vi "(Delta)^2_RH_v2 - Copy.vi"() -> ()   [LabVIEW 2019]
uses:
  <vilib>/Analysis/baseanly.llb/Mean (DBL).vi
  Components/DeltaRamp_globals.vi
  Components/B_Globals.vi
  Components/Global 2.vi
  <vilib>/Analysis/NI_AALBase.lvlib
panel:
  out "Arm 2":bool
  out "Arm 1":bool
  in  "Graphing":string(combo)
  in  "I_2":dbl
  out "T 3":cluster{"X":dbl[], "Y":dbl[]}[](graph)=[{"X"=[1.6944000000000004, 1.6942999999999993, 1.6944, 1.6942999999999993, 1.6942000000000002, 1.6943, 1.6941999999999995, 1.6943, 1.6942000000000002, 1.6943, 1.6944, 1.6942000000000006, 1.6942999999999993, 1.6944, 1.6942999999999988, 1.6942000000000002, 1.6942999999999993, 1.6942000000000002, 1.6940999999999997, 1.6942000000000002, 1.6944000000000008, 1.6945, 1.6944000000000008, 1.6942999999999993, 1.6944000000000008, 1.6942999999999988, 1.6944000000000004, 1.694299999999999, 1.6945, 1.6945999999999999, 1.6945, 1.6944000000000012, 1.694299999999999, 1.6944, 1.6945, 1.6944000000000008, 1.6945000000000006, 1.6946000000000003, 1.6944999999999995, 1.6945999999999999, 1.6944000000000004, 1.6945, 1.6945999999999999, 1.6945, 1.6944, 1.6945000000000017, 1.6946000000000003, 1.6947000000000005, 1.6948000000000003, 1.6949000000000003, 1.6948000000000003, 1.6947000000000008, 1.6946000000000008, 1.6947000000000005, 1.6948000000000005, 1.6947000000000003, 1.6946, 1.6947000000000008, 1.6945999999999999, 1.6947000000000005, 1.6946000000000006, 1.6947000000000008, 1.6948000000000003, 1.6946999999999992, 1.6948000000000003, 1.6947000000000005, 1.6948000000000005, 1.6949000000000003, 1.6948000000000005, 1.694899999999999, 1.6951, 1.695, 1.6949000000000003, 1.6948000000000003, 1.694899999999999, 1.695, 1.6948999999999992, 1.6948000000000003, 1.6947000000000008, 1.6949000000000003, 1.695, 1.6949000000000003, 1.695, 1.6949000000000003, 1.6948000000000003, 1.6949000000000003, 1.6948000000000003, 1.6949000000000003, 1.695, 1.6951, 1.6952, 1.6951, 1.6952, 1.6951, 1.695, 1.6948000000000003, 1.6949000000000003, 1.695], "Y"=[nan, nan, nan, nan, nan, nan, nan, nan, nan, nan, nan, nan, nan, nan, nan, nan, nan, nan, nan, nan, nan, nan, nan, nan, nan, nan, nan, nan, nan, nan, nan, nan, nan, nan, nan, nan, nan, nan, nan, nan, nan, nan, nan, nan, nan, nan, nan, nan, nan, nan, nan, nan, nan, nan, nan, nan, nan, nan, nan, nan, nan, nan, nan, nan, nan, nan, nan, nan, nan, nan, nan, nan, nan, nan, nan, nan, nan, nan, nan, nan, nan, nan, nan, nan, nan, nan, nan, nan, nan, nan, nan, nan, nan, nan, nan, nan, nan, nan]}, {"X"=[1.6944000000000004, 1.6942999999999993, 1.6944, 1.6942999999999993, 1.6942000000000002, 1.6943, 1.6941999999999995, 1.6943, 1.6942000000000002, 1.6943, 1.6944, 1.6942000000000006, 1.6942999999999993, 1.6944, 1.6942999999999988, 1.6942000000000002, 1.6942999999999993, 1.6942000000000002, 1.6940999999999997, 1.6942000000000002, 1.6944000000000008, 1.6945, 1.6944000000000008, 1.6942999999999993, 1.6944000000000008, 1.6942999999999988, 1.6944000000000004, 1.694299999999999, 1.6945, 1.6945999999999999, 1.6945, 1.6944000000000012, 1.694299999999999, 1.6944, 1.6945, 1.6944000000000008, 1.6945000000000006, 1.6946000000000003, 1.6944999999999995, 1.6945999999999999, 1.6944000000000004, 1.6945, 1.6945999999999999, 1.6945, 1.6944, 1.6945000000000017, 1.6946000000000003, 1.6947000000000005, 1.6948000000000003, 1.6949000000000003, 1.6948000000000003, 1.6947000000000008, 1.6946000000000008, 1.6947000000000005, 1.6948000000000005, 1.6947000000000003, 1.6946, 1.6947000000000008, 1.6945999999999999, 1.6947000000000005, 1.6946000000000006, 1.6947000000000008, 1.6948000000000003, 1.6946999999999992, 1.6948000000000003, 1.6947000000000005, 1.6948000000000005, 1.6949000000000003, 1.6948000000000005, 1.694899999999999, 1.6951, 1.695, 1.6949000000000003, 1.6948000000000003, 1.694899999999999, 1.695, 1.6948999999999992, 1.6948000000000003, 1.6947000000000008, 1.6949000000000003, 1.695, 1.6949000000000003, 1.695, 1.6949000000000003, 1.6948000000000003, 1.6949000000000003, 1.6948000000000003, 1.6949000000000003, 1.695, 1.6951, 1.6952, 1.6951, 1.6952, 1.6951, 1.695, 1.6948000000000003, 1.6949000000000003, 1.695], "Y"=[19.228962826666663, 19.229748019999995, 19.227549399999997, 19.232509233333335, 19.230370125, 19.231082114285716, 19.231533643749998, 19.2332894875, 19.234548728000004, 19.23138665, 19.23452267142857, 19.233269309999994, 19.2297025, 19.228221342857143, 19.230086174193545, 19.2305463125, 19.22998058125, 19.234866695833333, 19.232316606250002, 19.2317453, 19.234343370833333, 19.232386587500002, 19.231900426086955, 19.23144366666667, 19.23149760833333, 19.229992476666673, 19.230156412500005, 19.23336701304348, 19.2296826625, 19.232198475, 19.2310109125, 19.231653921794866, 19.228340475000003, 19.2295796875, 19.229462228571432, 19.2302099, 19.22956034666667, 19.233207449999995, 19.23203613684211, 19.232299549999997, 19.2309091125, 19.229504266666666, 19.230617525, 19.230744125, 19.231113187500004, 19.22967935322581, 19.230101100000002, 19.230308512500002, 19.228578285714285, 19.233646177777775, 19.231167942857144, 19.23003209333333, 19.23084153157895, 19.22980882222222, 19.23070347608696, 19.227994165217392, 19.230754216666664, 19.229694923529415, 19.23029495, 19.229152924999998, 19.231262049999998, 19.23127544, 19.231315600000002, 19.230833448717952, 19.229475299999997, 19.23220135, 19.229062404918036, 19.230352887500004, 19.23155630625, 19.23113153225807, 19.234514033333337, 19.23535129285714, 19.23361205, 19.232085249999997, 19.232065674999998, 19.230572292857143, 19.230861596666667, 19.2296080625, 19.231095506666673, 19.230930925, 19.230720785714286, 19.230639773333333, 19.231475349999997, 19.23118514, 19.2300918125, 19.232860700000003, 19.2284774875, 19.2328781875, 19.2326205, 19.230885100000002, 19.231523024999998, 19.229335787500002, 19.231723528571425, 19.231652535294117, 19.2325406, 19.22911017142857, 19.23088324375, 19.231545675]}] caption="XY Graph"
  out "T 2":cluster{"X":dbl[], "Y":dbl[]}[](graph)=[{"X"=[1.6944000000000004, 1.6942999999999993, 1.6944, 1.6942999999999993, 1.6942000000000002, 1.6943, 1.6941999999999995, 1.6943, 1.6942000000000002, 1.6943, 1.6944, 1.6942000000000006, 1.6942999999999993, 1.6944, 1.6942999999999988, 1.6942000000000002, 1.6942999999999993, 1.6942000000000002, 1.6940999999999997, 1.6942000000000002, 1.6944000000000008, 1.6945, 1.6944000000000008, 1.6942999999999993, 1.6944000000000008, 1.6942999999999988, 1.6944000000000004, 1.694299999999999, 1.6945, 1.6945999999999999, 1.6945, 1.6944000000000012, 1.694299999999999, 1.6944, 1.6945, 1.6944000000000008, 1.6945000000000006, 1.6946000000000003, 1.6944999999999995, 1.6945999999999999, 1.6944000000000004, 1.6945, 1.6945999999999999, 1.6945, 1.6944, 1.6945000000000017, 1.6946000000000003, 1.6947000000000005, 1.6948000000000003, 1.6949000000000003, 1.6948000000000003, 1.6947000000000008, 1.6946000000000008, 1.6947000000000005, 1.6948000000000005, 1.6947000000000003, 1.6946, 1.6947000000000008, 1.6945999999999999, 1.6947000000000005, 1.6946000000000006, 1.6947000000000008, 1.6948000000000003, 1.6946999999999992, 1.6948000000000003, 1.6947000000000005, 1.6948000000000005, 1.6949000000000003, 1.6948000000000005, 1.694899999999999, 1.6951, 1.695, 1.6949000000000003, 1.6948000000000003, 1.694899999999999, 1.695, 1.6948999999999992, 1.6948000000000003, 1.6947000000000008, 1.6949000000000003, 1.695, 1.6949000000000003, 1.695, 1.6949000000000003, 1.6948000000000003, 1.6949000000000003, 1.6948000000000003, 1.6949000000000003, 1.695, 1.6951, 1.6952, 1.6951, 1.6952, 1.6951, 1.695, 1.6948000000000003, 1.6949000000000003, 1.695], "Y"=[nan, nan, nan, nan, nan, nan, nan, nan, nan, nan, nan, nan, nan, nan, nan, nan, nan, nan, nan, nan, nan, nan, nan, nan, nan, nan, nan, nan, nan, nan, nan, nan, nan, nan, nan, nan, nan, nan, nan, nan, nan, nan, nan, nan, nan, nan, nan, nan, nan, nan, nan, nan, nan, nan, nan, nan, nan, nan, nan, nan, nan, nan, nan, nan, nan, nan, nan, nan, nan, nan, nan, nan, nan, nan, nan, nan, nan, nan, nan, nan, nan, nan, nan, nan, nan, nan, nan, nan, nan, nan, nan, nan, nan, nan, nan, nan, nan, nan]}, {"X"=[1.6944000000000004, 1.6942999999999993, 1.6944, 1.6942999999999993, 1.6942000000000002, 1.6943, 1.6941999999999995, 1.6943, 1.6942000000000002, 1.6943, 1.6944, 1.6942000000000006, 1.6942999999999993, 1.6944, 1.6942999999999988, 1.6942000000000002, 1.6942999999999993, 1.6942000000000002, 1.6940999999999997, 1.6942000000000002, 1.6944000000000008, 1.6945, 1.6944000000000008, 1.6942999999999993, 1.6944000000000008, 1.6942999999999988, 1.6944000000000004, 1.694299999999999, 1.6945, 1.6945999999999999, 1.6945, 1.6944000000000012, 1.694299999999999, 1.6944, 1.6945, 1.6944000000000008, 1.6945000000000006, 1.6946000000000003, 1.6944999999999995, 1.6945999999999999, 1.6944000000000004, 1.6945, 1.6945999999999999, 1.6945, 1.6944, 1.6945000000000017, 1.6946000000000003, 1.6947000000000005, 1.6948000000000003, 1.6949000000000003, 1.6948000000000003, 1.6947000000000008, 1.6946000000000008, 1.6947000000000005, 1.6948000000000005, 1.6947000000000003, 1.6946, 1.6947000000000008, 1.6945999999999999, 1.6947000000000005, 1.6946000000000006, 1.6947000000000008, 1.6948000000000003, 1.6946999999999992, 1.6948000000000003, 1.6947000000000005, 1.6948000000000005, 1.6949000000000003, 1.6948000000000005, 1.694899999999999, 1.6951, 1.695, 1.6949000000000003, 1.6948000000000003, 1.694899999999999, 1.695, 1.6948999999999992, 1.6948000000000003, 1.6947000000000008, 1.6949000000000003, 1.695, 1.6949000000000003, 1.695, 1.6949000000000003, 1.6948000000000003, 1.6949000000000003, 1.6948000000000003, 1.6949000000000003, 1.695, 1.6951, 1.6952, 1.6951, 1.6952, 1.6951, 1.695, 1.6948000000000003, 1.6949000000000003, 1.695], "Y"=[19.228962826666663, 19.229748019999995, 19.227549399999997, 19.232509233333335, 19.230370125, 19.231082114285716, 19.231533643749998, 19.2332894875, 19.234548728000004, 19.23138665, 19.23452267142857, 19.233269309999994, 19.2297025, 19.228221342857143, 19.230086174193545, 19.2305463125, 19.22998058125, 19.234866695833333, 19.232316606250002, 19.2317453, 19.234343370833333, 19.232386587500002, 19.231900426086955, 19.23144366666667, 19.23149760833333, 19.229992476666673, 19.230156412500005, 19.23336701304348, 19.2296826625, 19.232198475, 19.2310109125, 19.231653921794866, 19.228340475000003, 19.2295796875, 19.229462228571432, 19.2302099, 19.22956034666667, 19.233207449999995, 19.23203613684211, 19.232299549999997, 19.2309091125, 19.229504266666666, 19.230617525, 19.230744125, 19.231113187500004, 19.22967935322581, 19.230101100000002, 19.230308512500002, 19.228578285714285, 19.233646177777775, 19.231167942857144, 19.23003209333333, 19.23084153157895, 19.22980882222222, 19.23070347608696, 19.227994165217392, 19.230754216666664, 19.229694923529415, 19.23029495, 19.229152924999998, 19.231262049999998, 19.23127544, 19.231315600000002, 19.230833448717952, 19.229475299999997, 19.23220135, 19.229062404918036, 19.230352887500004, 19.23155630625, 19.23113153225807, 19.234514033333337, 19.23535129285714, 19.23361205, 19.232085249999997, 19.232065674999998, 19.230572292857143, 19.230861596666667, 19.2296080625, 19.231095506666673, 19.230930925, 19.230720785714286, 19.230639773333333, 19.231475349999997, 19.23118514, 19.2300918125, 19.232860700000003, 19.2284774875, 19.2328781875, 19.2326205, 19.230885100000002, 19.231523024999998, 19.229335787500002, 19.231723528571425, 19.231652535294117, 19.2325406, 19.22911017142857, 19.23088324375, 19.231545675]}] caption="XY Graph"
  in  "Clear Paths":bool
  out "Remote Inherit Path":path=path "C:/User Data/hlb54/210307/RH_T=35p00K.txt"
  out "Remote Directory":path=path "C:/User Data/hlb54/210307"
  out "Last Saved":path=path "C:/User Data/gy251/20210308 Nb2p5-EuS30-Nb3_C/Rxx_9-10-11-12/RT_10uA_1.txt"
  out "Remote_Save_String [This is the important one!]":string="RH_T=35p00K.txt"
  in  "L1 ID":string="56A"
  in  "D1 ID":string="GY1C"
  out "R2":dbl=19.2284241
  in  "D2_use":bool=TRUE
  in  "D1_use":bool
  in  "D2":refnum<visa-resource-name>="GPIB1::22::INSTR" caption="Back"
  in  "Front":refnum<visa-resource-name>="GPIB1::20::INSTR"
  out "B_set [T]":dbl=3.0
  in  "Reading Delay [ms]":i32=20 min=5
  in  "RW Delay":i32=5
  out "Exec Time [ms]":u32=39
  in  "B/T":bool=TRUE
  in  "Smart Avs":bool=TRUE
  in  "Points":dbl=1.0
  out "PpP":dbl=8.0
  in  "Combo Box":string(combo)="Temp"
  in  "Save":bool
  in  "Abort":bool
  out "B [T]":dbl=2.98877
  in  "Arm":bool
  in  "Measure":bool
  in  "I_1":dbl=5e-05
  out "T":cluster{"X":dbl[], "Y":dbl[]}[](graph)=[{"X"=[1.6944000000000004, 1.6942999999999993, 1.6944, 1.6942999999999993, 1.6942000000000002, 1.6943, 1.6941999999999995, 1.6943, 1.6942000000000002, 1.6943, 1.6944, 1.6942000000000006, 1.6942999999999993, 1.6944, 1.6942999999999988, 1.6942000000000002, 1.6942999999999993, 1.6942000000000002, 1.6940999999999997, 1.6942000000000002, 1.6944000000000008, 1.6945, 1.6944000000000008, 1.6942999999999993, 1.6944000000000008, 1.6942999999999988, 1.6944000000000004, 1.694299999999999, 1.6945, 1.6945999999999999, 1.6945, 1.6944000000000012, 1.694299999999999, 1.6944, 1.6945, 1.6944000000000008, 1.6945000000000006, 1.6946000000000003, 1.6944999999999995, 1.6945999999999999, 1.6944000000000004, 1.6945, 1.6945999999999999, 1.6945, 1.6944, 1.6945000000000017, 1.6946000000000003, 1.6947000000000005, 1.6948000000000003, 1.6949000000000003, 1.6948000000000003, 1.6947000000000008, 1.6946000000000008, 1.6947000000000005, 1.6948000000000005, 1.6947000000000003, 1.6946, 1.6947000000000008, 1.6945999999999999, 1.6947000000000005, 1.6946000000000006, 1.6947000000000008, 1.6948000000000003, 1.6946999999999992, 1.6948000000000003, 1.6947000000000005, 1.6948000000000005, 1.6949000000000003, 1.6948000000000005, 1.694899999999999, 1.6951, 1.695, 1.6949000000000003, 1.6948000000000003, 1.694899999999999, 1.695, 1.6948999999999992, 1.6948000000000003, 1.6947000000000008, 1.6949000000000003, 1.695, 1.6949000000000003, 1.695, 1.6949000000000003, 1.6948000000000003, 1.6949000000000003, 1.6948000000000003, 1.6949000000000003, 1.695, 1.6951, 1.6952, 1.6951, 1.6952, 1.6951, 1.695, 1.6948000000000003, 1.6949000000000003, 1.695], "Y"=[nan, nan, nan, nan, nan, nan, nan, nan, nan, nan, nan, nan, nan, nan, nan, nan, nan, nan, nan, nan, nan, nan, nan, nan, nan, nan, nan, nan, nan, nan, nan, nan, nan, nan, nan, nan, nan, nan, nan, nan, nan, nan, nan, nan, nan, nan, nan, nan, nan, nan, nan, nan, nan, nan, nan, nan, nan, nan, nan, nan, nan, nan, nan, nan, nan, nan, nan, nan, nan, nan, nan, nan, nan, nan, nan, nan, nan, nan, nan, nan, nan, nan, nan, nan, nan, nan, nan, nan, nan, nan, nan, nan, nan, nan, nan, nan, nan, nan]}, {"X"=[1.6944000000000004, 1.6942999999999993, 1.6944, 1.6942999999999993, 1.6942000000000002, 1.6943, 1.6941999999999995, 1.6943, 1.6942000000000002, 1.6943, 1.6944, 1.6942000000000006, 1.6942999999999993, 1.6944, 1.6942999999999988, 1.6942000000000002, 1.6942999999999993, 1.6942000000000002, 1.6940999999999997, 1.6942000000000002, 1.6944000000000008, 1.6945, 1.6944000000000008, 1.6942999999999993, 1.6944000000000008, 1.6942999999999988, 1.6944000000000004, 1.694299999999999, 1.6945, 1.6945999999999999, 1.6945, 1.6944000000000012, 1.694299999999999, 1.6944, 1.6945, 1.6944000000000008, 1.6945000000000006, 1.6946000000000003, 1.6944999999999995, 1.6945999999999999, 1.6944000000000004, 1.6945, 1.6945999999999999, 1.6945, 1.6944, 1.6945000000000017, 1.6946000000000003, 1.6947000000000005, 1.6948000000000003, 1.6949000000000003, 1.6948000000000003, 1.6947000000000008, 1.6946000000000008, 1.6947000000000005, 1.6948000000000005, 1.6947000000000003, 1.6946, 1.6947000000000008, 1.6945999999999999, 1.6947000000000005, 1.6946000000000006, 1.6947000000000008, 1.6948000000000003, 1.6946999999999992, 1.6948000000000003, 1.6947000000000005, 1.6948000000000005, 1.6949000000000003, 1.6948000000000005, 1.694899999999999, 1.6951, 1.695, 1.6949000000000003, 1.6948000000000003, 1.694899999999999, 1.695, 1.6948999999999992, 1.6948000000000003, 1.6947000000000008, 1.6949000000000003, 1.695, 1.6949000000000003, 1.695, 1.6949000000000003, 1.6948000000000003, 1.6949000000000003, 1.6948000000000003, 1.6949000000000003, 1.695, 1.6951, 1.6952, 1.6951, 1.6952, 1.6951, 1.695, 1.6948000000000003, 1.6949000000000003, 1.695], "Y"=[19.228962826666663, 19.229748019999995, 19.227549399999997, 19.232509233333335, 19.230370125, 19.231082114285716, 19.231533643749998, 19.2332894875, 19.234548728000004, 19.23138665, 19.23452267142857, 19.233269309999994, 19.2297025, 19.228221342857143, 19.230086174193545, 19.2305463125, 19.22998058125, 19.234866695833333, 19.232316606250002, 19.2317453, 19.234343370833333, 19.232386587500002, 19.231900426086955, 19.23144366666667, 19.23149760833333, 19.229992476666673, 19.230156412500005, 19.23336701304348, 19.2296826625, 19.232198475, 19.2310109125, 19.231653921794866, 19.228340475000003, 19.2295796875, 19.229462228571432, 19.2302099, 19.22956034666667, 19.233207449999995, 19.23203613684211, 19.232299549999997, 19.2309091125, 19.229504266666666, 19.230617525, 19.230744125, 19.231113187500004, 19.22967935322581, 19.230101100000002, 19.230308512500002, 19.228578285714285, 19.233646177777775, 19.231167942857144, 19.23003209333333, 19.23084153157895, 19.22980882222222, 19.23070347608696, 19.227994165217392, 19.230754216666664, 19.229694923529415, 19.23029495, 19.229152924999998, 19.231262049999998, 19.23127544, 19.231315600000002, 19.230833448717952, 19.229475299999997, 19.23220135, 19.229062404918036, 19.230352887500004, 19.23155630625, 19.23113153225807, 19.234514033333337, 19.23535129285714, 19.23361205, 19.232085249999997, 19.232065674999998, 19.230572292857143, 19.230861596666667, 19.2296080625, 19.231095506666673, 19.230930925, 19.230720785714286, 19.230639773333333, 19.231475349999997, 19.23118514, 19.2300918125, 19.232860700000003, 19.2284774875, 19.2328781875, 19.2326205, 19.230885100000002, 19.231523024999998, 19.229335787500002, 19.231723528571425, 19.231652535294117, 19.2325406, 19.22911017142857, 19.23088324375, 19.231545675]}] caption="XY Graph"
  in  "Reset":bool
  out "Spl T [K]":dbl=1.6949
  out "R1 [Ohm]":dbl=nan
  # "Use?"
  # "Armed?"
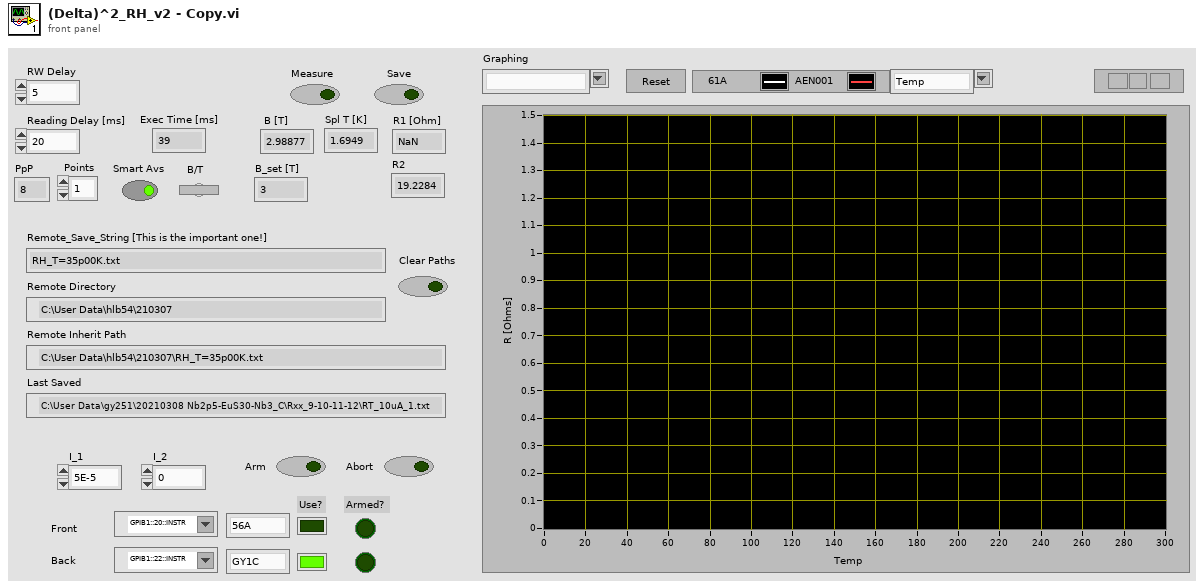
[diagram p1: front panel]
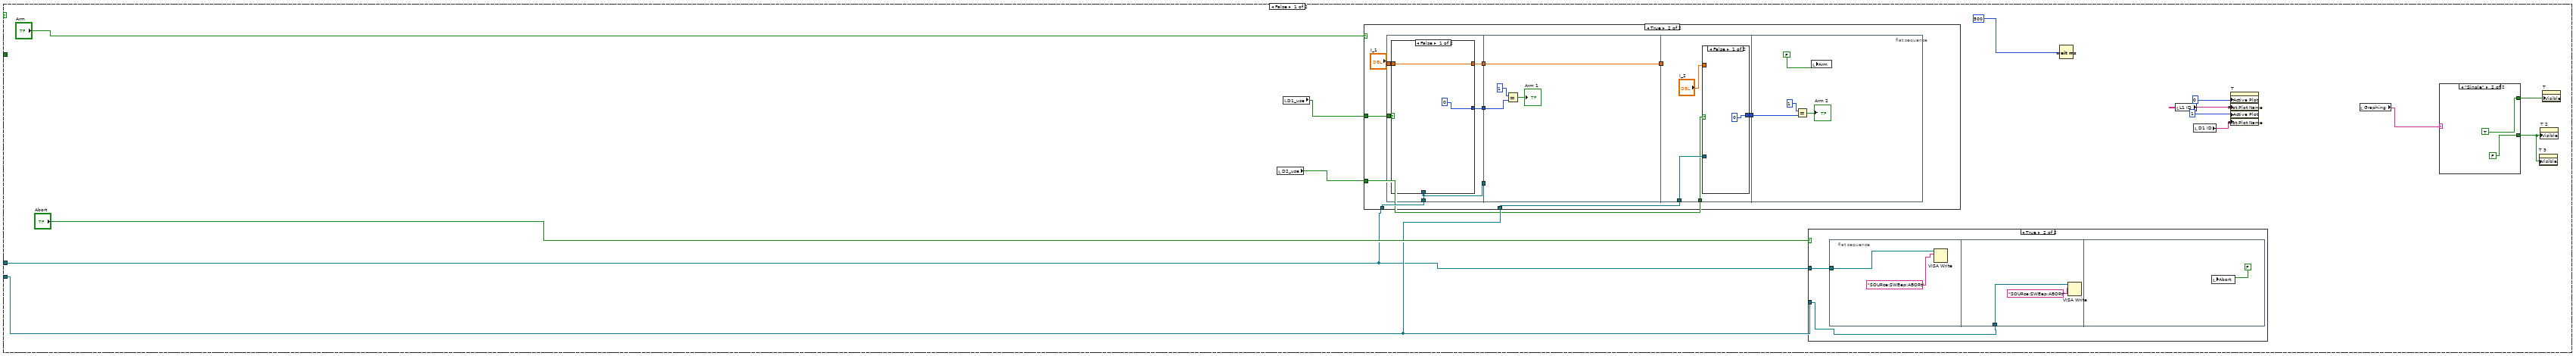
[diagram p2: hidden frame]
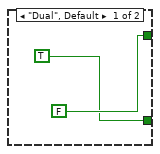
[diagram p3: hidden frame]
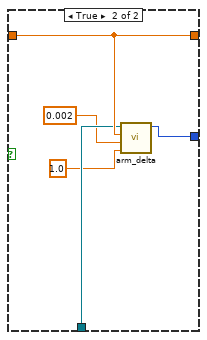
[diagram p6: hidden frame]
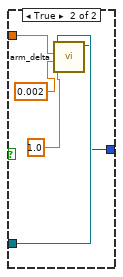
[diagram p7: hidden frame]
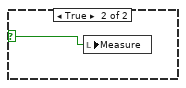
[diagram p8: hidden frame]
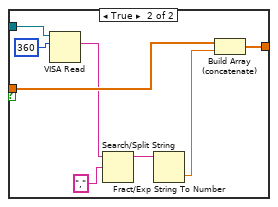
[diagram p13: hidden frame]
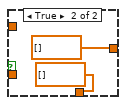
[diagram p14: hidden frame]
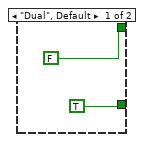
[diagram p15: hidden frame]
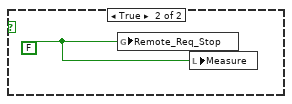
[diagram p17: hidden frame]
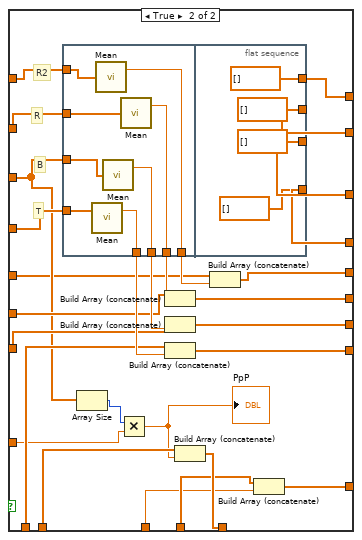
[diagram p18: hidden frame]
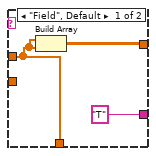
[diagram p19: hidden frame]
diagram:
  # "D2"
  # "D1"
  n1 = VISA Clear(VISA resource name="D2") -> (VISA resource name out=w3:refnum<visa-resource-name>)  [unwired: 1 in, 1 out]
  n2 = VISA Clear(VISA resource name="Front") -> (VISA resource name out=w1:refnum<visa-resource-name>)  [unwired: 1 in, 1 out]
  n3 = while {
    tunnel: w1 -> [w6]
    tunnel: w3 -> [w5]
    stop <- FALSE stop-if-true
    # "Short T"
    # "Short B"
    n4 = global read "DeltaRamp_globals.vi" "Remote_Measure"() -> (w7:bool)
    n5 = Or(x="Measure", y=w7) -> (x .or. y?=w9:bool)
    n6 = case shown="True" w9 {
      tunnel: w7 -> [_ w78]
      tunnel: w6 -> [w21 w77]
      tunnel: w5 -> [w22 w76]
      frame False {
        n7 = local read "D2_use"() -> (w19:bool)
        n8 = local read "D1_use"() -> (w20:bool)
        n9 = case shown="True" "Arm" {
          tunnel: w22 -> [_ w44]
          tunnel: w21 -> [_ w43]
          tunnel: w20 -> [_ w42]
          tunnel: w19 -> [_ w41]
          frame False {
          }
          frame True {
            n10 = flat-sequence {
              tunnel: [w50] -> w40
              tunnel: "I_1" -> [w49]
              tunnel: w43 -> [w47]
              tunnel: w42 -> [w48]
              tunnel: [w47] -> w38
              tunnel: [w46] -> w37
              tunnel: w40 -> [w61]
              tunnel: [w61] -> w39
              tunnel: w38 -> [_]
              tunnel: w37 -> [w59]
              tunnel: w39 -> [_]
              tunnel: w44 -> [w65]
              tunnel: w41 -> [w64]
              tunnel: [w62] -> w36
              tunnel: w36 -> [w73]
              frame #0 {
                n11 = case shown="False" w48 {
                  tunnel: [w52 w57] -> w50
                  tunnel: w49 -> [w52 w57]
                  tunnel: w47 -> [_ w56]
                  tunnel: [0 w53] -> w46
                  frame False {
                  }
                  frame True {
                    n12 = call "arm_delta.vi"("Compliance [V]"=1.0, "DELAY [sec]"=0.002, "I-HIGH [A]"=w57, "Keithley"=w56) -> ("number"=w53:i32)  [unwired: 7 in]
                  }
                }
              }
              frame #1 {
                n13 = Equal?(x=1, y=w59) -> (x = y?=→"Arm 1":bool)
              }
              frame #2 {
                n14 = case shown="False" w64 {
                  tunnel: "I_2" -> [_ w71]
                  tunnel: w65 -> [_ w68]
                  tunnel: [0 w67] -> w62
                  frame False {
                  }
                  frame True {
                    n15 = call "arm_delta.vi"("Compliance [V]"=1.0, "DELAY [sec]"=0.002, "I-HIGH [A]"=w71, "Keithley"=w68) -> ("number"=w67:i32)  [unwired: 7 in]
                  }
                }
              }
              frame #3 {
                n16 = Equal?(x=1, y=w73) -> (x = y?=→"Arm 2":bool)
                n17 = local write "Arm"(FALSE) -> ()
              }
            }
          }
        }
        n18 = case shown="True" "Abort" {
          tunnel: w22 -> [_ w30]
          tunnel: w21 -> [_ w29]
          frame False {
          }
          frame True {
            n19 = flat-sequence {
              tunnel: w29 -> [w31]
              tunnel: w30 -> [w33]
              frame #0 {
                n20 = VISA Write(VISA resource name=w31, write buffer="SOURce:SWEep:ABORt") -> ()  [unwired: 1 in, 3 out]
              }
              frame #1 {
                n21 = VISA Write(VISA resource name=w33, write buffer="SOURce:SWEep:ABORt") -> ()  [unwired: 1 in, 3 out]
              }
              frame #2 {
                n22 = local write "Abort"(FALSE) -> ()
              }
            }
          }
        }
        n23 = Wait (ms)(milliseconds to wait=500) -> ()  [unwired: 1 out]
        n24 = local read "L1 ID"() -> (w14:string)
        n25 = local read "D1 ID"() -> (w12:string)
        n26 = property on="T" class="XYGraph (strict)"("Active Plot"=0, "Plot.Plot Name"=w14, "Active Plot"=1, "Plot.Plot Name"=w12) -> ()  [unwired: 2 in, 2 out]
        n27 = local read "Graphing"() -> (w16:string)
        n28 = case shown="\"Single\"" w16 {
          tunnel: [FALSE TRUE] -> w18
          tunnel: [TRUE FALSE] -> w17
          frame "Dual", Default {
          }
          frame "Single" {
          }
        }
        n29 = property on="T 3" class="XYGraph (strict)"("Visible"=w17) -> ()  [unwired: 2 in, 2 out]
        n30 = property on="T 2" class="XYGraph (strict)"("Visible"=w17) -> ()  [unwired: 2 in, 2 out]
        n31 = property on="T" class="XYGraph (strict)"("Visible"=w18) -> ()  [unwired: 2 in, 2 out]
      }
      frame True {
        # "Ramp=False?"
        n32 = case shown="False" w78 {
          selector: w78 -> [_ w79]
          frame False {
          }
          frame True {
            n33 = local write "Measure"(w79) -> ()
          }
        }
        n34 = while {
          shift-right: [w139] -> _
          shift-left: _ -> [w145]
          shift-right: [w155] -> _
          shift-left: _ -> [w159]
          shift-right: [w153] -> _
          shift-left: _ -> [w164]
          shift-right: [w138] -> _
          shift-left: _ -> [w148]
          shift-right: [w140] -> _
          shift-left: _ -> [w152]
          shift-right: [w154] -> _
          shift-left: _ -> [w167]
          shift-right: [w173] -> _
          shift-left: _ -> [w174]
          shift-right: [w176] -> _
          shift-left: _ -> [w177]
          shift-right: [w123] -> _
          shift-left: _ -> [w127]
          tunnel: w77 -> [w120]
          tunnel: w76 -> [w119]
          shift-right: [w108] -> _
          shift-left: _ -> [w112]
          shift-right: [w106] -> _
          shift-left: _ -> [w104]
          stop <- w129 stop-if-true
          # "R2"
          n35 = global write "DeltaRamp_globals.vi" "Remote_Measure"(FALSE) -> ()
          n36 = flat-sequence {
            tunnel: w177 -> [w192]
            tunnel: [w190] -> w176
            tunnel: w167 -> [w189]
            tunnel: [w189] -> w166
            tunnel: w164 -> [w188]
            tunnel: [w188] -> w162
            tunnel: w159 -> [w187]
            tunnel: [w187] -> w158
            tunnel: w152 -> [w186]
            tunnel: [w186] -> w150
            tunnel: [w185] -> w149
            tunnel: w148 -> [w185]
            tunnel: [w184] -> w146
            tunnel: w145 -> [w184]
            tunnel: [w183] -> w128
            tunnel: w127 -> [w183]
            tunnel: w120 -> [w182]
            tunnel: w119 -> [w181]
            tunnel: [w182] -> w118
            tunnel: [w181] -> w117
            tunnel: [w180] -> w113
            tunnel: w112 -> [w180]
            tunnel: [w179] -> w105
            tunnel: w104 -> [w179]
            tunnel: w166 -> [w206]
            tunnel: [w206] -> w101
            tunnel: [w205] -> w99
            tunnel: w162 -> [w205]
            tunnel: [w204] -> w97
            tunnel: w158 -> [w204]
            tunnel: [w203] -> w95
            tunnel: w150 -> [w203]
            tunnel: w149 -> [w202]
            tunnel: [w202] -> w93
            tunnel: w146 -> [w201]
            tunnel: [w201] -> w91
            tunnel: w128 -> [w200]
            tunnel: [w200] -> w89
            tunnel: w118 -> [w199]
            tunnel: w117 -> [w198]
            tunnel: [w199] -> w87
            tunnel: [w198] -> w85
            tunnel: w113 -> [w197]
            tunnel: [w197] -> w83
            tunnel: w105 -> [w196]
            tunnel: [w196] -> w81
            tunnel: w101 -> [w218]
            tunnel: [w218] -> w100
            tunnel: w99 -> [w217]
            tunnel: [w217] -> w98
            tunnel: w97 -> [w216]
            tunnel: [w216] -> w96
            tunnel: w95 -> [w215]
            tunnel: [w215] -> w94
            tunnel: w93 -> [w214]
            tunnel: [w214] -> w92
            tunnel: w91 -> [w213]
            tunnel: [w213] -> w90
            tunnel: w89 -> [w212]
            tunnel: [w212] -> w88
            tunnel: w87 -> [w211]
            tunnel: [w211] -> w86
            tunnel: w85 -> [w210]
            tunnel: [w210] -> w84
            tunnel: w83 -> [w209]
            tunnel: [w209] -> w82
            tunnel: w81 -> [w208]
            tunnel: [w208] -> w80
            tunnel: [w235] -> w171
            tunnel: [w234] -> w169
            tunnel: w100 -> [w233]
            tunnel: [w233] -> w165
            tunnel: [w232] -> w163
            tunnel: w98 -> [w232]
            tunnel: w96 -> [w231]
            tunnel: [w231] -> w157
            tunnel: [w230] -> w151
            tunnel: w94 -> [w230]
            tunnel: [w229] -> w147
            tunnel: w92 -> [w229]
            tunnel: [w228] -> w144
            tunnel: w90 -> [w228]
            tunnel: [w227] -> w126
            tunnel: w88 -> [w227]
            tunnel: [w226] -> w122
            tunnel: [w225] -> w116
            tunnel: w86 -> [w225]
            tunnel: [w224] -> w115
            tunnel: w84 -> [w224]
            tunnel: w82 -> [w223]
            tunnel: [w223] -> w110
            tunnel: [w222] -> w103
            tunnel: w80 -> [w222]
            tunnel: [w256] -> w175
            tunnel: w174 -> [w256]
            tunnel: [w239] -> w172
            tunnel: w171 -> [w255]
            tunnel: [w255] -> w170
            tunnel: w169 -> [w254]
            tunnel: [w254] -> w168
            tunnel: w165 -> [w253]
            tunnel: w163 -> [w252]
            tunnel: [w253] -> w161
            tunnel: [w252] -> w160
            tunnel: w157 -> [w251]
            tunnel: [w251] -> w156
            tunnel: w151 -> [w250]
            tunnel: w147 -> [w249]
            tunnel: w144 -> [w248]
            tunnel: [w250] -> w143
            tunnel: [w249] -> w142
            tunnel: [w248] -> w141
            tunnel: ["Points"] -> w137
            tunnel: w126 -> [w246]
            tunnel: [w246] -> w125
            tunnel: w122 -> [w245]
            tunnel: [w245] -> w121
            tunnel: w116 -> [w241]
            tunnel: w115 -> [w242]
            tunnel: [w236] -> w114
            tunnel: [w238] -> w111
            tunnel: w110 -> [w238]
            tunnel: w103 -> [w237]
            tunnel: [w237] -> w102
            tunnel: w175 -> [w403]
            tunnel: w172 -> [w395]
            tunnel: w170 -> [w394]
            tunnel: w168 -> [w390]
            tunnel: w161 -> [w399]
            tunnel: w160 -> [w393]
            tunnel: w156 -> [w398]
            tunnel: w143 -> [w382]
            tunnel: w142 -> [w381]
            tunnel: w141 -> [w380]
            tunnel: w137 -> [w386]
            tunnel: [w387] -> w136
            tunnel: [w396] -> w135
            tunnel: [w392] -> w134
            tunnel: [w391] -> w133
            tunnel: [w362] -> w132
            tunnel: [w389] -> w131
            tunnel: [w388] -> w130
            tunnel: w125 -> [w383]
            tunnel: [w385] -> w124
            tunnel: w121 -> [w379]
            tunnel: w114 -> [w375]
            tunnel: w111 -> [w378]
            tunnel: [w376] -> w109
            tunnel: [w367] -> w107
            tunnel: w102 -> [w373]
            tunnel: [w613] -> w138
            tunnel: [w614] -> w139
            tunnel: [w615] -> w140
            tunnel: [w616] -> w153
            tunnel: [w617] -> w154
            tunnel: [w618] -> w155
            tunnel: [w619] -> w173
            tunnel: w136 -> [w619]
            tunnel: w135 -> [w618]
            tunnel: w134 -> [w617]
            tunnel: w133 -> [w616]
            tunnel: w132 -> [w615]
            tunnel: w131 -> [w614]
            tunnel: w130 -> [w613]
            tunnel: w124 -> [w611]
            tunnel: [w611] -> w123
            tunnel: [w610] -> w108
            tunnel: w109 -> [w610]
            tunnel: w107 -> [w609]
            tunnel: [w609] -> w106
            frame #0 {
              n37 = Tick Count (ms)() -> (millisecond timer value=w190:u32)
              n38 = Subtract(x=w190, y=w192) -> (x-y=→"Exec Time [ms]":u32)
            }
            frame #1 {
              n39 = global read "DeltaRamp_globals.vi" "Remote_Save_Directory"() -> (→"Remote Directory":path)
              n40 = global read "DeltaRamp_globals.vi" "Remote_Save_String"() -> (w194:string)
              n41 = global read "DeltaRamp_globals.vi" "Remote_Ramp_Path"() -> (→"Remote Inherit Path":path)
              n42 = local write "Remote_Save_String [This is the important one!]"(w194) -> ()
            }
            frame #2 {
              n43 = case shown="True" "Clear Paths" {
                frame False {
                }
                frame True {
                  n44 = flat-sequence {
                    frame #0 {
                      w219 = path ""
                      n45 = global write "DeltaRamp_globals.vi" "Remote_Save_Directory"(w219) -> ()
                      n46 = global write "DeltaRamp_globals.vi" "Remote_Save_String"("") -> ()
                      n47 = global write "DeltaRamp_globals.vi" "Remote_Ramp_Path"(w219) -> ()
                    }
                    frame #1 {
                      n48 = local write "Clear Paths"(FALSE) -> ()
                    }
                  }
                }
              }
            }
            frame #3 {
              n49 = global read "Global 2.vi" "SampleTemp"() -> (w234:dbl)
              "Spl T [K]" <- w234
              n50 = global read "B_Globals.vi" "G_B_set[T]"() -> (w226:dbl)
              "B_set [T]" <- w226
              n51 = global read "B_Globals.vi" "B [T]"() -> (w235:dbl)
              "B [T]" <- w235
            }
            frame #4 {
              # "R2"
              # "Bset"
              # "Points"
              # "Short R"
              # "New T"
              # "New B"
              # "Short T"
              # "Short B"
              # "New R"
              n52 = for {
                N: "Points" -> [_]
                shift-right: [w268] -> w257
                shift-left: _ -> [w272]
                tunnel: "D2_use" -> [w261]
                tunnel: "D1_use" -> [w271]
                tunnel: w242 -> [w260]
                tunnel: w241 -> [w270]
                shift-right: [w263] -> w240
                shift-left: _ -> [w267]
                i -> [w273]
                n53 = Wait (ms)(milliseconds to wait=0) -> ()  [unwired: 1 out]
                n54 = Equal?(x=0, y=w273) -> (x = y?=w275:bool)
                n55 = case shown="False" w275 {
                  tunnel: [w347 dbl[] [] ("Numeric")] -> w269
                  tunnel: w272 -> [w347 _]
                  tunnel: w267 -> [w346 _]
                  tunnel: [w346 dbl[] [] ("Numeric")] -> w259
                  frame False {
                  }
                  frame True {
                  }
                }
                n56 = flat-sequence {
                  tunnel: w271 -> [w286]
                  tunnel: w270 -> [w295]
                  tunnel: w269 -> [w294]
                  tunnel: "RW Delay" -> [w292]
                  tunnel: [w293] -> w265
                  tunnel: [w286] -> w262
                  tunnel: w261 -> [w283]
                  tunnel: w260 -> [w282]
                  tunnel: w259 -> [w281]
                  tunnel: [w278] -> w258
                  tunnel: [w345] -> w268
                  tunnel: w265 -> [w345]
                  tunnel: w261 -> [_]
                  tunnel: w260 -> [_]
                  tunnel: w259 -> [_]
                  tunnel: "RW Delay" -> [_]
                  tunnel: [w344] -> w263
                  tunnel: w262 -> [_]
                  tunnel: w258 -> [w344]
                  frame #0 {
                    n57 = flat-sequence {
                      tunnel: w295 -> [w296]
                      tunnel: [w296] -> w291
                      tunnel: w291 -> [w297]
                      tunnel: [w297] -> w290
                      tunnel: [w302] -> w289
                      tunnel: w290 -> [w303]
                      tunnel: w286 -> [w301]
                      tunnel: [w301] -> w284
                      tunnel: w283 -> [w299]
                      tunnel: w282 -> [w300]
                      tunnel: [w299] -> w280
                      tunnel: [w298] -> w277
                      tunnel: [w316] -> w288
                      tunnel: w289 -> [w316]
                      tunnel: w292 -> [w315]
                      tunnel: [w314] -> w285
                      tunnel: w284 -> [w314]
                      tunnel: w280 -> [w313]
                      tunnel: [w313] -> w279
                      tunnel: w277 -> [w312]
                      tunnel: [w312] -> w276
                      tunnel: w288 -> [w324]
                      tunnel: w294 -> [w323]
                      tunnel: [w322] -> w287
                      tunnel: w285 -> [w321]
                      tunnel: w281 -> [w320]
                      tunnel: w279 -> [w319]
                      tunnel: [w318] -> w278
                      tunnel: w276 -> [w317]
                      tunnel: [w343] -> w293
                      tunnel: w287 -> [w343]
                      frame #0 {
                      }
                      frame #1 {
                      }
                      frame #2 {
                        n58 = case shown="True" w299 {
                          tunnel: w300 -> [w304 w307]
                          tunnel: [w304 w306] -> w298
                          frame False {
                          }
                          frame True {
                            n59 = VISA Write(VISA resource name=w307, write buffer="SENS:DATA:FRESh?") -> (VISA resource name out=w306:refnum<visa-resource-name>)  [unwired: 1 in, 2 out]
                          }
                        }
                        n60 = case shown="True" w301 {
                          tunnel: w303 -> [w308 w311]
                          tunnel: [w308 w310] -> w302
                          frame False {
                          }
                          frame True {
                            n61 = VISA Write(VISA resource name=w311, write buffer="SENS:DATA:FRESh?") -> (VISA resource name out=w310:refnum<visa-resource-name>)  [unwired: 1 in, 2 out]
                          }
                        }
                      }
                      frame #3 {
                        n62 = Wait (ms)(milliseconds to wait=w315) -> ()  [unwired: 1 out]
                      }
                      frame #4 {
                        n63 = case shown="True" w319 {
                          tunnel: w320 -> [w325 w332]
                          tunnel: [w325 w331] -> w318
                          tunnel: w317 -> [_ w326]
                          frame False {
                          }
                          frame True {
                            n64 = VISA Read(VISA resource name=w326, byte count=u32 360) -> (read buffer=w329:string)  [unwired: 1 in, 3 out]
                            n65 = Search/Split String(string=w329, search string/char (-)=",") -> (substring before match=w328:string)  [unwired: 1 in, 2 out]
                            n66 = Fract/Exp String To Number(string=w328) -> (number=w327:dbl)  [unwired: 1 in, 3 out]
                            n67 = Build Array (concatenate)(w332, w327) -> (w331:dbl[])
                          }
                        }
                        n68 = case shown="False" w321 {
                          tunnel: w324 -> [_ w341]
                          tunnel: w323 -> [w334 w340]
                          tunnel: [w334 w339] -> w322
                          frame False {
                          }
                          frame True {
                            n69 = VISA Read(VISA resource name=w341, byte count=u32 360) -> (read buffer=w337:string)  [unwired: 1 in, 3 out]
                            n70 = Search/Split String(string=w337, search string/char (-)=",") -> (substring before match=w336:string)  [unwired: 1 in, 2 out]
                            n71 = Fract/Exp String To Number(string=w336) -> (number=w335:dbl)  [unwired: 1 in, 3 out]
                            n72 = Build Array (concatenate)(w340, w335) -> (w339:dbl[])
                          }
                        }
                      }
                      frame #5 {
                      }
                    }
                  }
                  frame #1 {
                  }
                }
              }
              n73 = call-poly <vilib>:"Mean.vi"("X"=w257) -> ("mean"=w239:dbl)  [unwired: 1 out]
              n74 = call-poly <vilib>:"Mean.vi"("X"=w240) -> ("mean"=w236:dbl)  [unwired: 1 out]
            }
            frame #5 {
              # "PpP"
              n75 = global read "DeltaRamp_globals.vi" "Remote_Ramp_Save"() -> (w413:bool)
              n76 = Delete From Array(array=w393) -> (deleted portion=w401:dbl)  [unwired: 2 in, 1 out]
              n77 = Delete From Array(array=w399) -> (deleted portion=w400:dbl)  [unwired: 2 in, 1 out]
              n78 = Or(x="Save", y=w413) -> (x .or. y?=w408:bool)
              n79 = case shown="True" w408 {
                tunnel: w413 -> [_ w499]
                tunnel: w403 -> [_ w498]
                tunnel: w383 -> [_ w494]
                tunnel: w382 -> [_ w497]
                tunnel: w381 -> [_ w496]
                tunnel: w380 -> [_ w495]
                tunnel: w373 -> [_ w493]
                tunnel: "Save" -> [_ w492]
                frame False {
                }
                frame True {
                  n80 = flat-sequence {
                    tunnel: w499 -> [w501]
                    tunnel: w498 -> [w520]
                    tunnel: w497 -> [w532]
                    tunnel: w496 -> [w526]
                    tunnel: w495 -> [w524]
                    tunnel: w494 -> [w518]
                    tunnel: w493 -> [w522]
                    tunnel: w492 -> [w586]
                    tunnel: [w587] -> w491
                    tunnel: w491 -> [_]
                    frame #0 {
                      # "BSet"
                      # "PpP"
                      # "D1"
                      # "L1"
                      # "T"
                      # "B"
                      n81 = global read "DeltaRamp_globals.vi" "Remote_Save_String"() -> (w506:string)
                      "Remote_Save_String [This is the important one!]" <- w506
                      n82 = call "Convert to Dynamic Data5"("Array"=w532) -> ("Dynamic Data Type"=w529:dynamicdata)  [unwired: 3 in]
                      n83 = call "Convert to Dynamic Data"("Array"=w520) -> ("Dynamic Data Type"=w528:dynamicdata)  [unwired: 3 in]
                      n84 = call "Convert to Dynamic Data4"("Array"=w524) -> ("Dynamic Data Type"=w530:dynamicdata)  [unwired: 3 in]
                      n85 = call "Convert to Dynamic Data3"("Array"=w526) -> ("Dynamic Data Type"=w531:dynamicdata)  [unwired: 3 in]
                      n86 = call "Convert to Dynamic Data10"("Array"=w522) -> ("Dynamic Data Type"=w521:dynamicdata)  [unwired: 3 in]
                      n87 = call "Convert to Dynamic Data11"("Array"=w520) -> ("Dynamic Data Type"=w519:dynamicdata)  [unwired: 3 in]
                      n88 = call "Convert to Dynamic Data9"("Array"=w524) -> ("Dynamic Data Type"=w523:dynamicdata)  [unwired: 3 in]
                      n89 = call "Convert to Dynamic Data8"("Array"=w526) -> ("Dynamic Data Type"=w525:dynamicdata)  [unwired: 3 in]
                      n90 = call "Convert to Dynamic Data7"("Array"=w518) -> ("Dynamic Data Type"=w527:dynamicdata)  [unwired: 3 in]
                      n91 = local read "D2_use"() -> (w504:bool)
                      n92 = global read "DeltaRamp_globals.vi" "Remote_Save_String"() -> (w508:string)
                      n93 = call "Convert to Dynamic Data12"("Array"=w518) -> ("Dynamic Data Type"=w517:dynamicdata)  [unwired: 3 in]
                      n94 = local read "D1_use"() -> (w516:bool)
                      n95 = global read "DeltaRamp_globals.vi" "Remote_Save_Directory"() -> (w511:path)
                      n96 = Merge Signals(w531, w530, w529, w528, w527) -> (w533:dynamicdata)
                      n97 = Merge Signals(w525, w523, w521, w519, w517) -> (w503:dynamicdata)
                      n98 = Equal?(x=w506, y="") -> (x = y?=w500:bool)
                      n99 = Concatenate Strings("D1 ID", "_", w508) -> (w509:string)
                      n100 = Concatenate Strings("L1 ID", "_", w506) -> (w513:string)
                      n101 = Build Path(base path=w511, name or relative path=w513) -> (appended path=w512:path)
                      n102 = Build Path(base path=w511, name or relative path=w509) -> (appended path=w502:path)
                      n103 = flat-sequence {
                        tunnel: w533 -> [w538]
                        tunnel: w500 -> [w537]
                        tunnel: w516 -> [w536]
                        tunnel: w501 -> [w535]
                        tunnel: w512 -> [w534]
                        tunnel: w504 -> [w564]
                        tunnel: w503 -> [w563]
                        tunnel: w502 -> [w562]
                        tunnel: w501 -> [w561]
                        tunnel: w500 -> [w560]
                        frame #0 {
                          n104 = case shown="True" w536 {
                            tunnel: w538 -> [_ w542]
                            tunnel: w537 -> [_ w541]
                            tunnel: w535 -> [_ w540]
                            tunnel: w534 -> [_ w539]
                            frame False {
                            }
                            frame True {
                              n105 = flat-sequence {
                                tunnel: w542 -> [w547]
                                tunnel: w541 -> [w546]
                                tunnel: [w545] -> w543
                                tunnel: w539 -> [w544]
                                tunnel: w543 -> [w554]
                                tunnel: w540 -> [w558]
                                frame #0 {
                                n106 = case shown="False" w546 {
                                tunnel: w547 -> [w550 w552]
                                tunnel: [w549 w551] -> w545
                                tunnel: w544 -> [w548 _]
                                frame False {
                                n107 = call "Write To Measurement File2"("Signals"=w550, "Filename"=w548) -> ("Filename Out"=w549:path)  [unwired: 15 in, 2 out]
                                }
                                frame True {
                                n108 = call "Write To Measurement File"("Signals"=w552, "Reset"=TRUE) -> ("Filename Out"=w551:path)  [unwired: 15 in, 2 out]
                                }
                                }
                                }
                                frame #1 {
                                w556 = path ""
                                n109 = call <vilib>:"Is Path and Not Empty.vi"("path"=w554) -> ("Is Path and Not Empty?"=w557:bool)  [unwired: 4 in]
                                n110 = local write "Last Saved"(w554) -> ()
                                n111 = global write "DeltaRamp_globals.vi" "Remote_Ramp_Path"(w556) -> ()
                                n112 = global write "DeltaRamp_globals.vi" "Remote_Save_String"("") -> ()
                                n113 = global write "DeltaRamp_globals.vi" "Remote_Save_Directory"(w556) -> ()
                                n114 = case shown="True" w558 {
                                tunnel: w557 -> [_ w559]
                                frame False {
                                }
                                frame True {
                                n115 = local write "Reset"(w559) -> ()
                                }
                                }
                                }
                                frame #2 {
                                }
                              }
                            }
                          }
                        }
                        frame #1 {
                          n116 = case shown="True" w564 {
                            tunnel: w563 -> [_ w568]
                            tunnel: w562 -> [_ w567]
                            tunnel: w561 -> [_ w566]
                            tunnel: w560 -> [_ w565]
                            frame False {
                            }
                            frame True {
                              n117 = flat-sequence {
                                tunnel: w568 -> [w573]
                                tunnel: w567 -> [w572]
                                tunnel: [w571] -> w569
                                tunnel: w565 -> [w570]
                                tunnel: w569 -> [w580]
                                tunnel: w566 -> [w584]
                                frame #0 {
                                n118 = case shown="False" w570 {
                                tunnel: w573 -> [w576 w578]
                                tunnel: w572 -> [w575 _]
                                tunnel: [w574 w577] -> w571
                                frame False {
                                n119 = call "Write To Measurement File3"("Signals"=w576, "Filename"=w575) -> ("Filename Out"=w574:path)  [unwired: 15 in, 2 out]
                                }
                                frame True {
                                n120 = call "Write To Measurement File4"("Signals"=w578, "Reset"=TRUE) -> ("Filename Out"=w577:path)  [unwired: 15 in, 2 out]
                                }
                                }
                                }
                                frame #1 {
                                w582 = path ""
                                n121 = call <vilib>:"Is Path and Not Empty.vi"("path"=w580) -> ("Is Path and Not Empty?"=w583:bool)  [unwired: 4 in]
                                n122 = local write "Last Saved"(w580) -> ()
                                n123 = global write "DeltaRamp_globals.vi" "Remote_Save_Directory"(w582) -> ()
                                n124 = global write "DeltaRamp_globals.vi" "Remote_Ramp_Path"(w582) -> ()
                                n125 = global write "DeltaRamp_globals.vi" "Remote_Save_String"("") -> ()
                                n126 = case shown="True" w584 {
                                tunnel: w583 -> [_ w585]
                                frame False {
                                }
                                frame True {
                                n127 = local write "Reset"(w585) -> ()
                                }
                                }
                                }
                                frame #2 {
                                }
                              }
                            }
                          }
                        }
                      }
                    }
                    frame #1 {
                      n128 = global write "DeltaRamp_globals.vi" "Remote_Skip"(w586) -> ()
                    }
                    frame #2 {
                      w587 = FALSE
                      n129 = global write "DeltaRamp_globals.vi" "Remote_Ramp_Save"(w587) -> ()
                      n130 = local write "Save"(w587) -> ()
                    }
                    frame #3 {
                    }
                  }
                }
              }
              n131 = Array Size(array=w393) -> (size(s)=w418:i32)
              n132 = Not Equal?(x=w401, y=w390) -> (x != y?=w419:bool)
              n133 = Not Equal?(x=w394, y=w400) -> (x != y?=w422:bool)
              n134 = Greater?(x=w418, y=1) -> (0:w421:bool)
              n135 = And(x=w421, y=w422) -> (x .and. y?=w423:bool)
              n136 = And(x=w421, y=w419) -> (x .and. y?=w424:bool)
              n137 = case shown="True" "B/T" {
                tunnel: w423 -> [w432 _]
                tunnel: w424 -> [_ w433]
                tunnel: [w432 w433] -> w425
                frame False {
                  # "B"
                }
                frame True {
                  # "T"
                }
              }
              n138 = Not(x="Smart Avs") -> (.not. x?=w415:bool)
              n139 = Or(x=w415, y=w425) -> (x .or. y?=w416:bool)
              n140 = case shown="False" w416 {
                tunnel: [w443 w472] -> w427
                tunnel: [w441 w471] -> w397
                tunnel: [w442 w458] -> w426
                tunnel: [w438 w469] -> w405
                tunnel: [w440 w468] -> w406
                tunnel: [w439 w466] -> w407
                tunnel: [w444 w464] -> w402
                tunnel: w403 -> [w444 w463]
                tunnel: w399 -> [w443 w454]
                tunnel: w393 -> [w442 w459]
                tunnel: w398 -> [w441 w460]
                tunnel: w382 -> [w440 w457]
                tunnel: w381 -> [w438 w456]
                tunnel: w380 -> [w439 w455]
                tunnel: w386 -> [_ w453]
                tunnel: w383 -> [w437 w452]
                tunnel: [w437 w451] -> w384
                tunnel: w379 -> [_ w450]
                tunnel: w378 -> [w436 w449]
                tunnel: [w436 w448] -> w377
                tunnel: [w435 w446] -> w374
                tunnel: w373 -> [w435 w445]
                frame False {
                }
                frame True {
                  # "R2"
                  # "T"
                  # "B"
                  # "R"
                  n141 = flat-sequence {
                    tunnel: [w479] -> w470
                    tunnel: [w478] -> w465
                    tunnel: [w480] -> w467
                    tunnel: w460 -> [w477]
                    tunnel: w454 -> [w476]
                    tunnel: w459 -> [w475]
                    tunnel: w449 -> [w474]
                    tunnel: [w473] -> w447
                    tunnel: [dbl[] []] -> w458
                    tunnel: [dbl[] []] -> w472
                    tunnel: [dbl[] []] -> w471
                    tunnel: [dbl[] []] -> w448
                    frame #0 {
                      n142 = call-poly <vilib>:"Mean.vi"("X"=w475) -> ("mean"=w480:dbl)  [unwired: 1 out]
                      n143 = call-poly <vilib>:"Mean.vi"("X"=w474) -> ("mean"=w473:dbl)  [unwired: 1 out]
                      n144 = call-poly <vilib>:"Mean.vi"("X"=w476) -> ("mean"=w479:dbl)  [unwired: 1 out]
                      n145 = call-poly <vilib>:"Mean.vi"("X"=w477) -> ("mean"=w478:dbl)  [unwired: 1 out]
                    }
                    frame #1 {
                    }
                  }
                  n146 = Array Size(array=w454) -> (size(s)=w462:i32)
                  n147 = Multiply(x=w462, y=w453) -> (x*y=w461:dbl)
                  "PpP" <- w461
                  n148 = Build Array (concatenate)(w457, w465) -> (w468:dbl[])
                  n149 = Build Array (concatenate)(w456, w470) -> (w469:dbl[])
                  n150 = Build Array (concatenate)(w455, w467) -> (w466:dbl[])
                  n151 = Build Array (concatenate)(w463, w461) -> (w464:dbl[])
                  n152 = Build Array (concatenate)(w445, w447) -> (w446:dbl[])
                  n153 = Build Array (concatenate)(w452, w450) -> (w451:dbl[])
                }
              }
              n154 = global read "DeltaRamp_globals.vi" "Remote_Reset"() -> (w409:bool)
              n155 = Or(x="Reset", y=w409) -> (x .or. y?=w411:bool)
              n156 = Build Array (concatenate)(w426, w390) -> (w391:dbl[])
              n157 = case shown="False" w411 {
                tunnel: w405 -> [w593 w602]
                tunnel: [w593 w601] -> w388
                tunnel: w407 -> [w592 w600]
                tunnel: [w592 w599] -> w389
                tunnel: [w591 w598] -> w362
                tunnel: w406 -> [w591 _]
                tunnel: [w590 w596] -> w387
                tunnel: w402 -> [w590 _]
                tunnel: [w589 w595] -> w385
                tunnel: w384 -> [w589 _]
                tunnel: w374 -> [w588 _]
                tunnel: [w588 w594] -> w367
                frame False {
                }
                frame True {
                  w597 = FALSE
                  n158 = flat-sequence {
                    tunnel: w602 -> [_]
                    tunnel: w600 -> [_]
                    tunnel: [dbl[] []] -> w599
                    tunnel: [dbl[] []] -> w601
                    tunnel: [dbl[] []] -> w598
                    tunnel: [dbl[] [] ("Numeric")] -> w596
                    tunnel: [dbl[] [] ("Numeric")] -> w595
                    tunnel: [dbl[] [] ("Numeric")] -> w594
                    frame #0 {
                    }
                  }
                  n159 = global write "DeltaRamp_globals.vi" "Remote_Reset"(w597) -> ()
                  n160 = local write "Reset"(w597) -> ()
                }
              }
              n161 = global read "DeltaRamp_globals.vi" "Remote_Req_Stop"() -> (w412:bool)
              n162 = Build Array (concatenate)(w427, w394) -> (w392:dbl[])
              n163 = Build Array (concatenate)(w397, w395) -> (w396:dbl[])
              n164 = Build Array (concatenate)(w377, w375) -> (w376:dbl[])
              n165 = case shown="\"Temp\"" "Combo Box" {
                tunnel: w389 -> [_ w489]
                tunnel: w388 -> [w486 _]
                tunnel: [w487 w490] -> w370
                tunnel: [w486 w489] -> w364
                tunnel: ["T" "K"] -> w350
                frame "Field", Default {
                  n166 = Build Array(w486, w486) -> (w487:dbl[][])
                }
                frame "Temp" {
                  n167 = Build Array(w489, w489) -> (w490:dbl[][])
                }
              }
              n168 = case shown="False" w412 {
                frame False {
                }
                frame True {
                  w434 = FALSE
                  n169 = global write "DeltaRamp_globals.vi" "Remote_Req_Stop"(w434) -> ()
                  n170 = local write "Measure"(w434) -> ()
                }
              }
              n171 = call "Convert to Dynamic Data15"("Array"=w364) -> ("Dynamic Data Type"=w363:dynamicdata)  [unwired: 3 in]
              n172 = call "Convert to Dynamic Data16"("Array"=w362) -> ("Dynamic Data Type"=w361:dynamicdata)  [unwired: 3 in]
              n173 = Build Array(w362, w367) -> (w372:dbl[][])
              n174 = call "Build XY Graph3"("Y Input"=w361, "X Input"=w363) -> ("XY Graph"=→"T 3":cluster{"X":dbl[], "Y":dbl[]}[])  [unwired: 8 in, 1 out]
              n175 = call "Convert to Dynamic Data14"("Array"=w364) -> ("Dynamic Data Type"=w365:dynamicdata)  [unwired: 3 in]
              n176 = call "Convert to Dynamic Data13"("Array"=w367) -> ("Dynamic Data Type"=w366:dynamicdata)  [unwired: 3 in]
              n177 = call "Convert to Dynamic Data6"("2D Array"=w370) -> ("Dynamic Data Type"=w369:dynamicdata)  [unwired: 3 in]
              n178 = call "Convert to Dynamic Data2"("2D Array"=w372) -> ("Dynamic Data Type"=w371:dynamicdata)  [unwired: 3 in]
              n179 = case shown="\"Single\"" "Graphing" {
                tunnel: [TRUE FALSE] -> w357
                tunnel: [FALSE TRUE] -> w356
                frame "Dual", Default {
                }
                frame "Single" {
                }
              }
              n180 = call "Build XY Graph2"("Y Input"=w371, "X Input"=w369) -> ("XY Graph"=→"T":cluster{"X":dbl[], "Y":dbl[]}[])  [unwired: 8 in, 1 out]
              n181 = call "Build XY Graph"("Y Input"=w366, "X Input"=w365) -> ("XY Graph"=→"T 2":cluster{"X":dbl[], "Y":dbl[]}[])  [unwired: 8 in, 1 out]
              n182 = local read "L1 ID"() -> (w353:string)
              n183 = local read "D1 ID"() -> (w352:string)
              n184 = property on="T" class="XYGraph (strict)"("Visible"=w356) -> ()  [unwired: 2 in, 2 out]
              n185 = property on="T 3" class="XYGraph (strict)"("Visible"=w357, "Plot.Plot Name"=w352, "XScale.NameLbl.Text"="Combo Box", "XScale.UnitLabel.Text"=w350) -> ()  [unwired: 2 in, 2 out]
              n186 = property on="T" class="XYGraph (strict)"("Active Plot"=0, "Plot.Plot Name"=w353, "Active Plot"=1, "Plot.Plot Name"=w352, "XScale.UnitLabel.Text"=w350, "XScale.NameLbl.Text"="Combo Box") -> ()  [unwired: 2 in, 2 out]
              n187 = property on="T 2" class="XYGraph (strict)"("Visible"=w357, "XScale.NameLbl.Text"="Combo Box", "Plot.Plot Name"=w353, "XScale.UnitLabel.Text"=w350) -> ()  [unwired: 2 in, 2 out]
              "R1 [Ohm]" <- w395
              "R2" <- w375
            }
            frame #6 {
              n188 = Wait (ms)(milliseconds to wait="Reading Delay [ms]") -> ()  [unwired: 1 out]
            }
          }
          n189 = local read "Measure"() -> (w129:bool)
        }
      }
    }
  }
